vi "Get Error Count Channels.vi"(8 "error in":errorcluster, 11 "Ballard MIL-STD-1553 custom device in":T2 format="%.0x") -> (0 "error out":errorcluster, 2 "error count channel refs":T1={"general protocol"=18446744073709551615, "improper number of words"=18446744073709551615, "Manchester"=18446744073709551615, "monitor"=18446744073709551615, "parity"=18446744073709551615, "unconfigured frames"=18446744073709551615, "word"=18446744073709551615, "wrong sync"=18446744073709551615} {"wrong sync" format="%.0x"; "word" format="%.0x"; "unconfigured frames" format="%.0x"; "parity" format="%.0x"; "monitor" format="%.0x"; "Manchester" format="%.0x"; "improper number of words" format="%.0x"; "general protocol" format="%.0x"}, 3 "Ballard MIL-STD-1553 custom device out":T2 format="%.0x", 4 "found?":bool)   [LabVIEW 2020, in "Ballard MIL-STD-1553 Scripting.lvlib"]
uses:
  Ballard MIL-STD-1553 Scripting.lvlib
  <vilib>/NI VeriStand/Custom Device API/Custom Device Item Ref.ctl
  Constants.vi
  <vilib>/NI VeriStand/Custom Device Tools/Custom Device Utility Library/NI VeriStand - Search for Item by GUID.vi
  <vilib>/NI VeriStand/Custom Device Tools/Custom Device Utility Library/NI VeriStand - Search for Item by Name.vi
  <vilib>/NI VeriStand/Custom Device Tools/Custom Device Utility Library/Custom Device Utility Library.lvlib
  <vilib>/NI VeriStand/Custom Device API/Custom Device API.lvlib
  Shared/Error Count Channel Refs.ctl
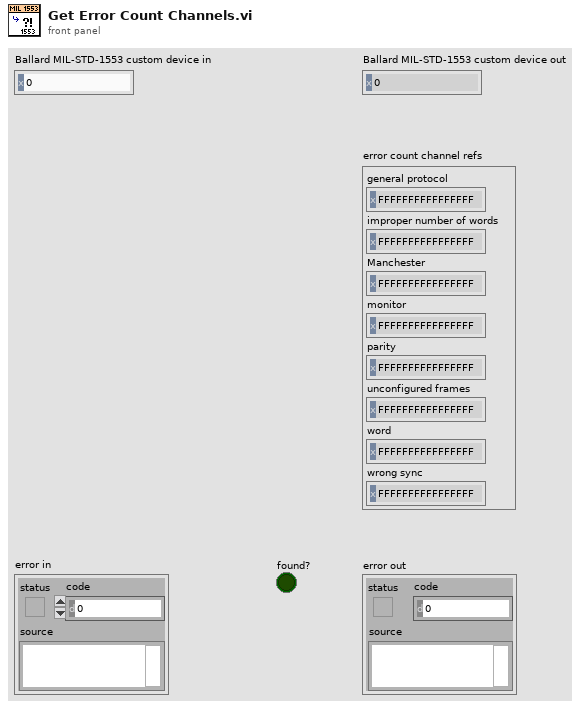
[diagram p1: front panel]
types:
  T1 = typedef "Error Count Channel Refs.ctl" = cluster{"general protocol":T2, "improper number of words":T2, "Manchester":T2, "monitor":T2, "parity":T2, "unconfigured frames":T2, "word":T2, "wrong sync":T2}
  T2 = typedef "Custom Device API.lvlib/Custom Device Item Ref.ctl" = u64
  T3 = cluster{"general protocol":T2, "improper number of words":T2, "Manchester":T2, "monitor":T2, "parity":T2, "unconfigured frames":T2, "word":T2, "wrong sync":T2}
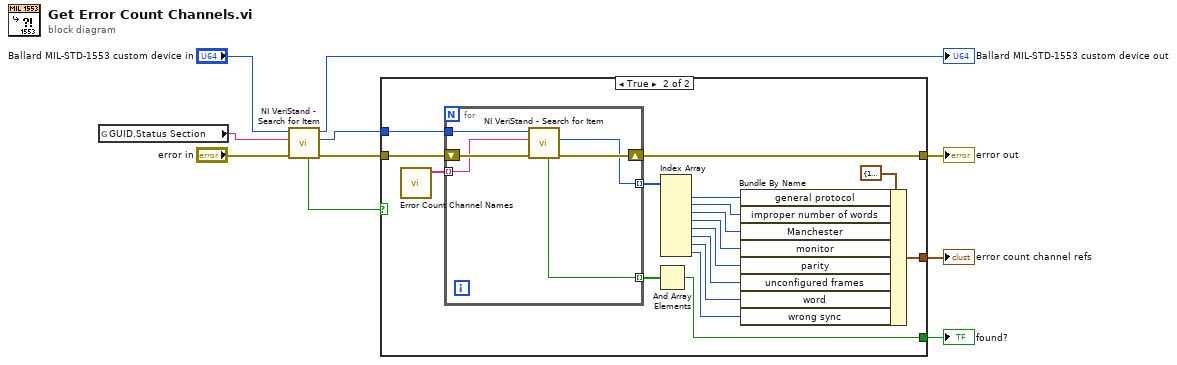
[diagram p0: block diagram]
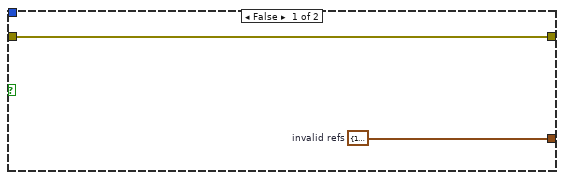
[diagram p2: hidden frame]
diagram:
  n1 = global read "Constants.vi" "GUID.Status Section"() -> (w3:string)
  n2 = call-poly <vilib>:"NI VeriStand - Search for Item.vi"("error in"="error in", "Item GUID"=w3, "Section Ref in"="Ballard MIL-STD-1553 custom device in") -> ("error out"=w4:errorcluster, "Item Ref"=w7:T2, "Section Ref out"=→"Ballard MIL-STD-1553 custom device out":T2, "Found"=w2:bool)  [unwired: 5 in]
  n3 = case shown="True" w2 {
    tunnel: [w12 w27] -> w10
    tunnel: [w11 w17] -> w9
    tunnel: w7 -> [_ w16]
    tunnel: w4 -> [w12 w15]
    tunnel: [_ w13] -> w1
    frame False {
      w11 = T3 {"general protocol"=18446744073709551615, "improper number of words"=18446744073709551615, "Manchester"=18446744073709551615, "monitor"=18446744073709551615, "parity"=18446744073709551615, "unconfigured frames"=18446744073709551615, "word"=18446744073709551615, "wrong sync"=18446744073709551615}  # invalid refs
    }
    frame True {
      n4 = call "Error Count Channel Names.vi"() -> ("error count channel names"=w29:string[])  [unwired: 11 in]
      n5 = for {
        shift-right: [w33] -> w27
        shift-left: w15 -> [w34]
        tunnel: w29 -> [w32] mode=indexing
        tunnel: [w31] -> w28 mode=indexing
        tunnel: w16 -> [w35]
        tunnel: [w30] -> w14 mode=indexing
        n6 = call-poly <vilib>:"NI VeriStand - Search for Item.vi"("error in"=w34, "Item Name"=w32, "Section Ref in"=w35) -> ("error out"=w33:errorcluster, "Item Ref"=w31:T2, "Found"=w30:bool)  [unwired: 5 in, 1 out]
      }
      n7 = And Array Elements(Boolean array=w14) -> (logical AND=w13:bool)
      n8 = Index Array(array=w28) -> (element #1=w25:T2, element #2=w24:T2, element #3=w23:T2, element #4=w22:T2, element #5=w21:T2, element #6=w20:T2, element #7=w19:T2, element #8=w18:T2)  [unwired: 8 in]
      n9 = Bundle By Name(cluster=T3 {"general protocol"=18446744073709551615, "improper number of words"=18446744073709551615, "Manchester"=18446744073709551615, "monitor"=18446744073709551615, "parity"=18446744073709551615, "unconfigured frames"=18446744073709551615, "word"=18446744073709551615, "wrong sync"=18446744073709551615} ("error count channel refs"), "general protocol"=w25, "improper number of words"=w24, "Manchester"=w23, "monitor"=w22, "parity"=w21, "unconfigured frames"=w20, "word"=w19, "wrong sync"=w18) -> (w17:T3)
    }
  }
  "error out" <- w10
  "error count channel refs" <- w9
  "found?" <- w1
